vi "test_UDP Write.vi"(8 "error in (no error)":errorcluster, 11 "TestCase in":refnum<class "Instrument Addon Ethernet Protocol Unit Tests.lvclass">) -> (0 "error out":errorcluster, 3 "TestCase out":refnum<class "Instrument Addon Ethernet Protocol Unit Tests.lvclass">)   [LabVIEW 2023, in "Instrument Addon Ethernet Protocol Unit Tests.lvclass"]
uses:
  Instrument Addon Ethernet Protocol Unit Tests.lvclass
  <vilib>/addons/_JKI Toolkits/VI Tester/TestCase.llb/TestCase.lvclass
  UDP/UDP.lvclass
  Listener/Listener.lvclass
  Listener/ListenerClassControls/Operation.ctl
  Constants.vi
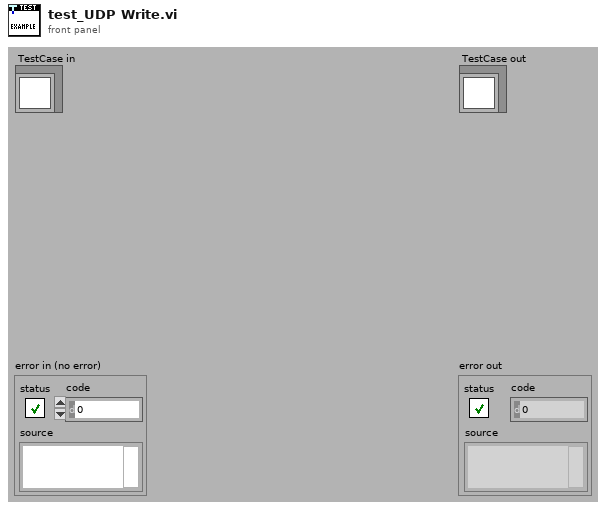
[diagram p1: front panel]
types:
  T1 = typedef "Listener.lvclass/Operation.ctl" = enum16{"Read", "Write"}
  T2 = typedef "Listener.lvclass/UDP Data Structure.ctl" = cluster{"UDP connection ID":refnum<k16>, "Local Address":string, "Local Port":u16, "Target IP Address":string, "Target Port":u16, "Data":string}
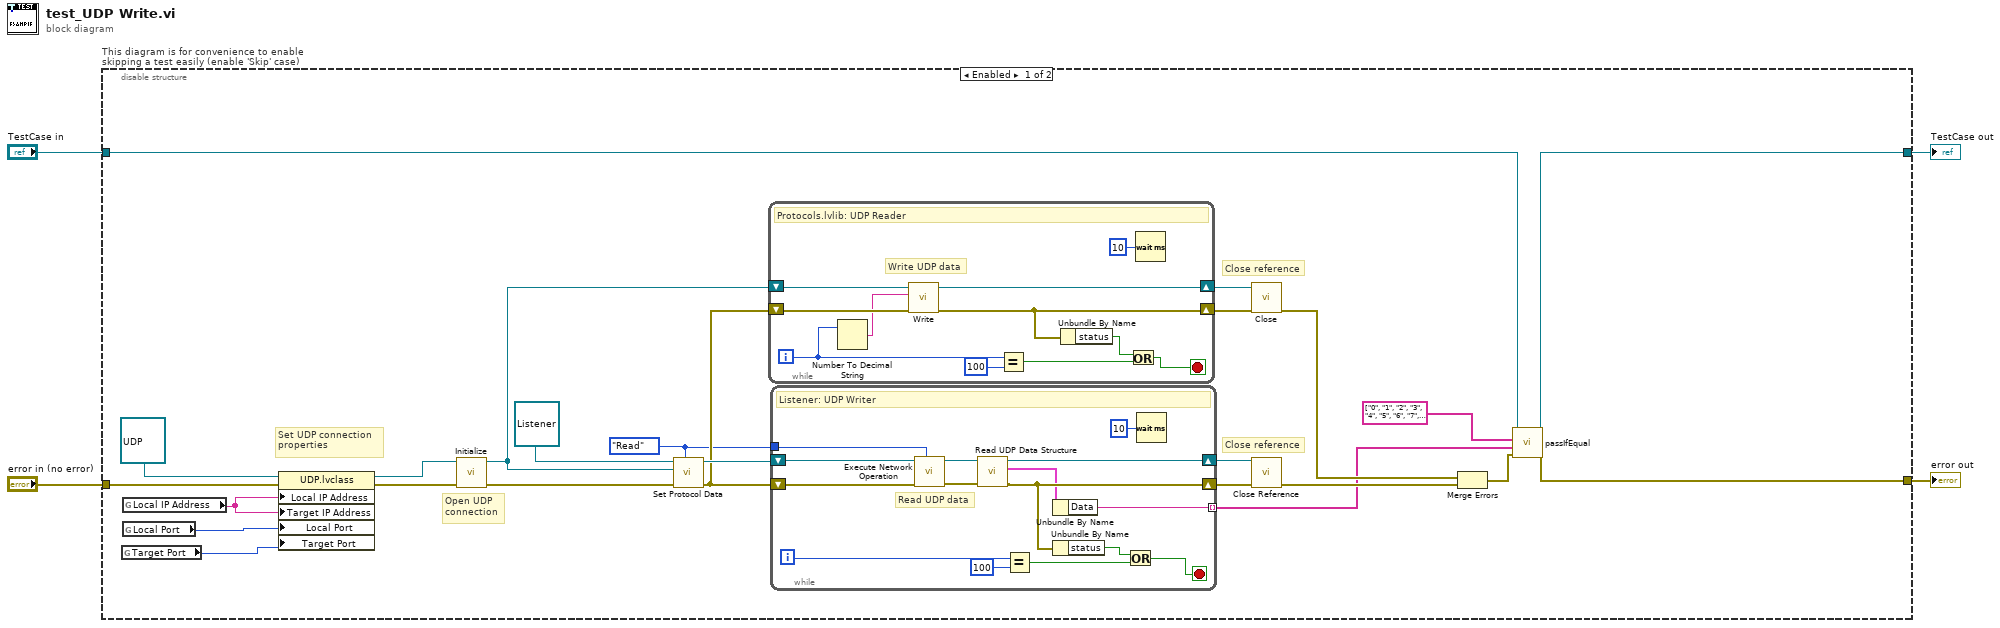
[diagram p0: block diagram]
diagram:
  n1 = disable-structure "This diagram is for convenience to enable skipping a test easily (enable 'Skip' case)" shown="Enabled" {
    disable-tunnel: "TestCase in" -> [w29 w59]
    disable-tunnel: [w28 w57] -> w1
    disable-tunnel: [w27 w58] -> w3
    disable-tunnel: "error in (no error)" -> [w25 w56]
    frame Enabled {
      w5 = Operation."Read" ("Operation")
      # "Close reference"
      # "Close reference"
      # "Open UDP \nconnection"
      # "Set UDP connection \nproperties"
      n2 = global read "Constants.vi" "Target Port"() -> (w6:u16)
      n3 = global read "Constants.vi" "Local IP Address"() -> (w8:string)
      n4 = global read "Constants.vi" "Local Port"() -> (w7:u16)
      n5 = property class="UDP.lvclass"(reference=refnum<class "UDP.lvclass"> refnum ("Protocols.lvlib:UDP.lvclass"), error in=w25, "Local IP Address"=w8, "Target IP Address"=w8, "Local Port"=w7, "Target Port"=w6) -> (reference out=w24:refnum<class "UDP.lvclass">, error out=w23:errorcluster)
      n6 = call-dynamic "Initialize.vi"("error in (no error)"=w23, "UDP in"=w24) -> ("error out"=w22:errorcluster, "UDP out"=w19:refnum<class "UDP.lvclass">)  [unwired: 8 in]
      n7 = call "Set Protocol Data.vi"("Operation"=w5, "error in (no error)"=w22, "Protocols.lvlib:Protocol Parent.lvclass"=w19, "Listener In.lvclass"=refnum<class "Listener.lvclass"> refnum ("Listener.lvclass")) -> ("error out"=w18:errorcluster, "Listener Out.lvclass"=w20:refnum<class "Listener.lvclass">)  [unwired: 6 in]
      n8 = while {
        shift-right: [w45] -> w15
        shift-left: w18 -> [w51]
        shift-right: [w49] -> w14
        shift-left: w19 -> [w50]
        i -> [w48]
        stop <- w52 stop-if-true
        # "Write UDP data"
        # "Protocols.lvlib: UDP Reader"
        n9 = Number To Decimal String(number=w48) -> (decimal integer string=w47:string)  [unwired: 1 in]
        n10 = call-dynamic "Write.vi"("error in (no error)"=w51, "String"=w47, "UDP in"=w50) -> ("error out"=w45:errorcluster, "UDP out"=w49:refnum<class "UDP.lvclass">)  [unwired: 7 in]
        n11 = Equal?(x=w48, y=100) -> (x = y?=w53:bool)
        n12 = Unbundle By Name(w45) -> ("status"=w46:bool)
        n13 = Or(x=w46, y=w53) -> (x .or. y?=w52:bool)
        n14 = Wait (ms)(milliseconds to wait=u32 10) -> ()  [unwired: 1 out]
      }
      n15 = while {
        shift-right: [w33] -> w11
        shift-left: w20 -> [w43]
        shift-right: [w34] -> w12
        shift-left: w18 -> [w44]
        tunnel: [w31] -> w9 mode=indexing
        tunnel: w5 -> [w30]
        i -> [w37]
        stop <- w38 stop-if-true
        # "Read UDP data"
        # "Listener: UDP Writer"
        n16 = call "Execute Network Operation.vi"("Operation"=w30, "error in (no error)"=w44, "Listener In.lvclass"=w43) -> ("error out"=w36:errorcluster, "Listener Out.lvclass"=w35:refnum<class "Listener.lvclass">)  [unwired: 7 in]
        n17 = call-dynamic "Read UDP Data Structure.vi"("error in (no error)"=w36, "Listener in"=w35) -> ("error out"=w34:errorcluster, "UDP Data Structure"=w32:T2, "Listener out"=w33:refnum<class "Listener.lvclass">)  [unwired: 7 in]
        n18 = Equal?(x=w37, y=100) -> (x = y?=w40:bool)
        n19 = Unbundle By Name(w32) -> ("Data"=w31:string)
        n20 = Unbundle By Name(w34) -> ("status"=w39:bool)
        n21 = Or(x=w39, y=w40) -> (x .or. y?=w38:bool)
        n22 = Wait (ms)(milliseconds to wait=u32 10) -> ()  [unwired: 1 out]
      }
      n23 = call-dynamic "Close.vi"("error in (no error)"=w15, "UDP in"=w14) -> ("error out"=w13:errorcluster)  [unwired: 8 in, 1 out]
      n24 = call "Close Reference.vi"("error in (no error)"=w12, "Listener In.lvclass"=w11) -> ("error out"=w10:errorcluster)  [unwired: 8 in, 1 out]
      n25 = Merge Errors(w13, w10) -> (w17:errorcluster)
      n26 = call-dynamic "passIfEqual.vi"("error in (no error)"=w17, "y"=w9, "x"=string[] ["0", "1", "2", "3", "4", "5", "6", "7", "8", "9", "10", "11", "12", "13", "14", "15", "16", "17", "18", "19", "20", "21", "22", "23", "24", "25", "26", "27", "28", "29", "30", "31", "32", "33", "34", "35", "36", "37", "38", "39", "40", "41", "42", "43", "44", "45", "46", "47", "48", "49", "50", "51", "52", "53", "54", "55", "56", "57", "58", "59", "60", "61", "62", "63", "64", "65", "66", "67", "68", "69", "70", "71", "72", "73", "74", "75", "76", "77", "78", "79", "80", "81", "82", "83", "84", "85", "86", "87", "88", "89", "90", "91", "92", "93", "94", "95", "96", "97", "98", "99", "100"] ("Array"), "TestCase in"=w29) -> ("error out"=w27:errorcluster, "TestCase out"=w28:refnum<class "Instrument Addon Ethernet Protocol Unit Tests.lvclass">)  [unwired: 6 in]
    }
    frame Disabled {
      # "skip test result while test is under development"
      n27 = call <vilib>:"skip.vi"("error in (no error)"=w56, "TestCase in"=w59) -> ("error out"=w58:errorcluster, "TestCase out"=w57:refnum<class "Instrument Addon Ethernet Protocol Unit Tests.lvclass">)  [unwired: 8 in]
    }
  }
  "error out" <- w3
  "TestCase out" <- w1
